vi "Export Image to Bmp File Or ClipBoard.vi"(7 "目标":enum32{"File", "Clipboard"}(ring), 8 "error in (no error)":errorcluster caption="错误输入（无错误）", 10 "路径":path, 11 "Table Ref In":refnum<vi>) -> (0 "error out":errorcluster caption="错误输出", 3 "Table Ref Out":refnum<vi>)   [LabVIEW 2012, in "Table Tool.lvlib"]
uses:
  Table Tool.lvlib
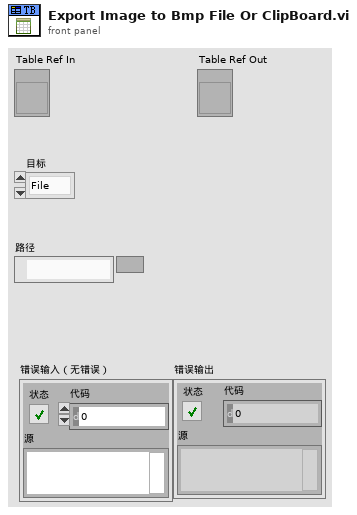
[diagram p1: front panel]
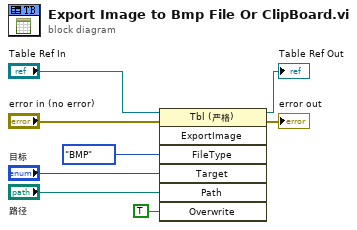
[diagram p0: block diagram]
diagram:
  n1 = invoke class="Tbl (严格)" method="ExportImage"(reference="Table Ref In", error in="error in (no error)", "FileType"=enum32{"BMP", "EPS", "EMF", "PICT"}."BMP" ("文件类型"), "Target"="目标", "Path"="路径", "Overwrite"=TRUE ("始终覆盖")) -> (reference out=→"Table Ref Out":refnum<vi>, error out=→"error out":errorcluster)  [unwired: 1 in, 5 out]
